vi "Calibration Verfiy new.vi"() -> ()   [LabVIEW 2011]
panel:
  out "error out 2":errorcluster
  out "StatusIsFalse 8":i16
  out "StatusIsFalse 7":i32
  out "StatusIsFalse 3":i16
  out "DONE?":bool
  out "Need More Pwr Reporting":i16
  out "Numeric 2":i32
  out "StatusIsFalse 6":i16
  out "StatusIsFalse 5":i16
  out "StatusIsFalse 4":i16
  out "StatusIsFalse 2":i16
  out "StatusIsFalse":i16
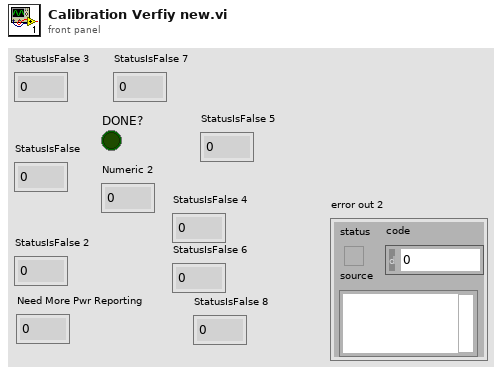
[diagram p1: front panel]
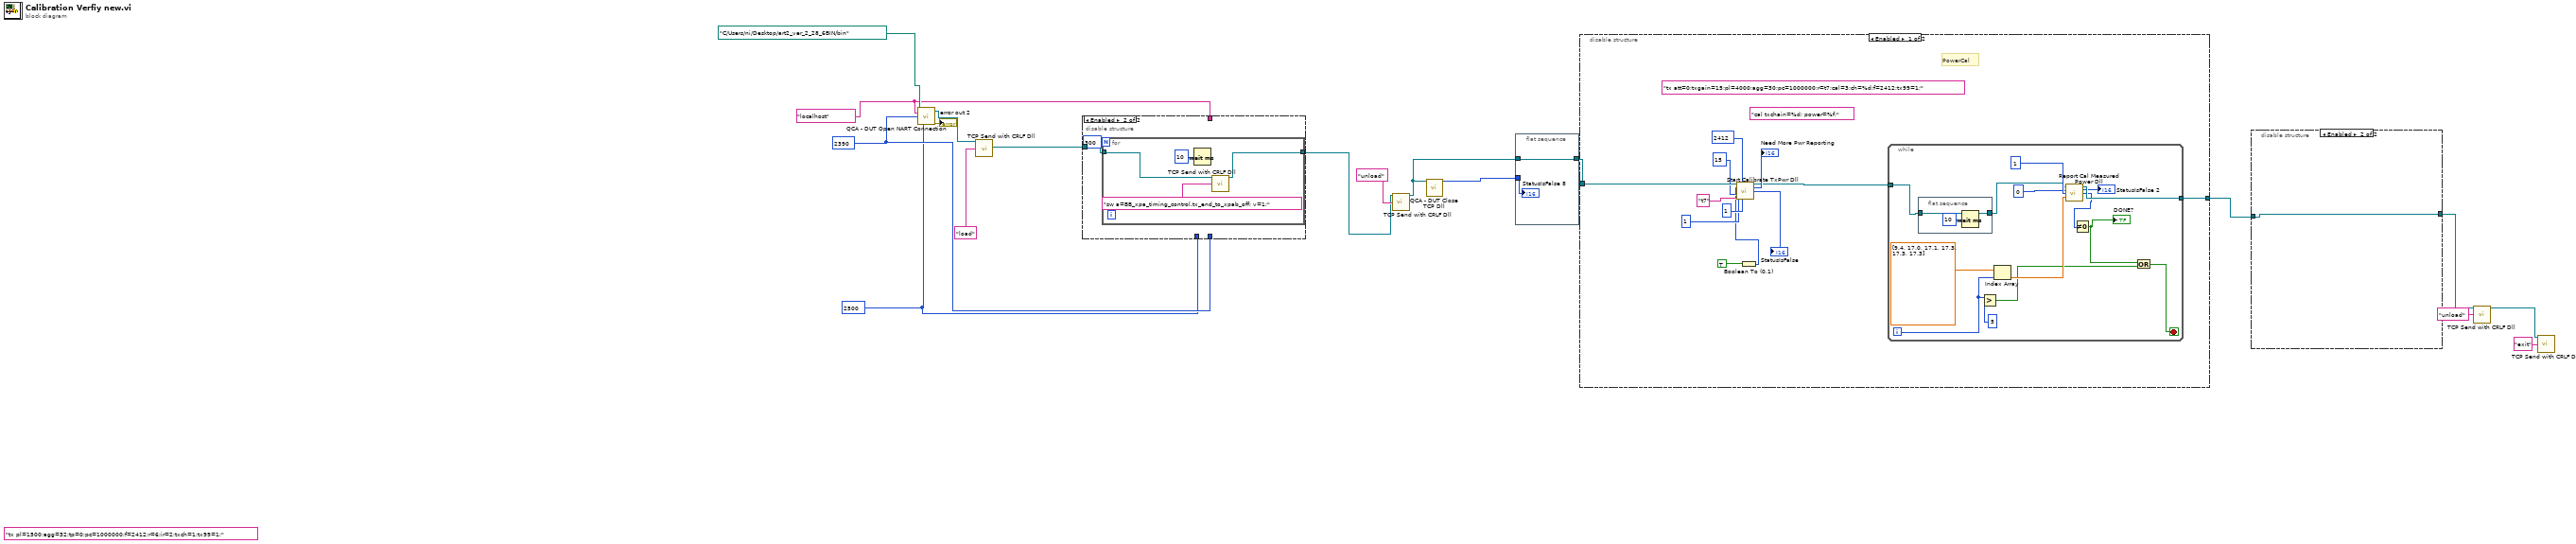
[diagram p0: block diagram]
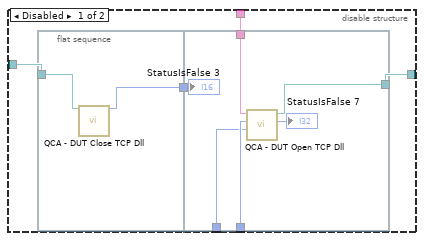
[diagram p2: hidden frame]
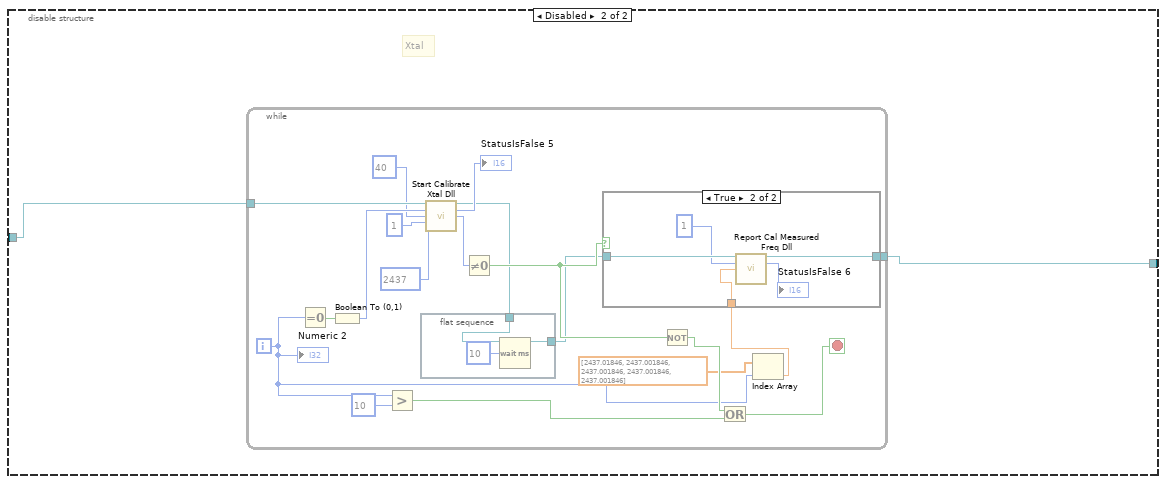
[diagram p3: hidden frame]
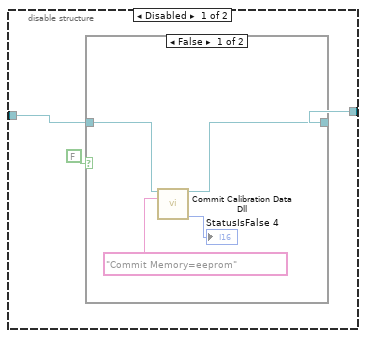
[diagram p5: hidden frame]
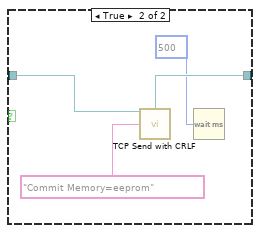
[diagram p6: hidden frame]
diagram:
  (unwired) "tx pl=1500;agg=32;tp=0;pc=1000000;f=2412;r=6;ir=2;txch=1;tx99=1;"
  w9 = 2500 ("Timeout (2500ms)")
  w10 = u32 2390 ("port (2390)")
  w11 = "localhost" ("IP Address (\"\": localhost)")
  n1 = call "QCA - DUT Open NART Connection.vi"("NART Directory"=path "C:/Users/ni/Desktop/art2_ver_2_28_6BIN/bin", "IP Address (\"\": localhost)"=w11, "port (2390)"=w10, "Timeout (2500ms)"=w9) -> ("NART TCP Connection"=w17:refnum<k5>, "error out"=→"error out 2":errorcluster)  [unwired: 10 in]
  n2 = call "TCP Send with CRLF Dll.vi"("CART TCP Connection"=w17, "CommandIn"="load") -> ("CART TCP Connection Out"=w4:refnum<k5>)  [unwired: 13 in]
  n3 = disable-structure shown="Enabled" {
    disable-tunnel: w4 -> [w23 w35]
    disable-tunnel: w11 -> [w22 _]
    disable-tunnel: w10 -> [w21 _]
    disable-tunnel: w9 -> [w20 _]
    disable-tunnel: [w19 w34] -> w1
    frame Disabled {
      n4 = flat-sequence {
        tunnel: w23 -> [w26]
        tunnel: [w25] -> w24
        tunnel: w22 -> [w32]
        tunnel: w21 -> [w31]
        tunnel: w20 -> [w30]
        tunnel: [w29] -> w19
        tunnel: w24 -> [w28]
        frame #0 {
          n5 = call "QCA - DUT Close TCP Dll.vi"("CART TCP Connection"=w26) -> ("StatusIsFalse"=w25:i16)  [unwired: 14 in]
        }
        frame #1 {
          n6 = call "QCA - DUT Open TCP Dll.vi"("Timeout (2500ms)"=w30, "port (2390)"=w31, "IP Address (\"\": localhost)"=w32) -> ("StatusIsFalse"=→"StatusIsFalse 7":i32, "NART TCP Connection"=w29:refnum<k5>)  [unwired: 7 in]
          "StatusIsFalse 3" <- w28
        }
      }
    }
    frame Enabled {
      n7 = for {
        N: 300 -> [_]
        tunnel: w35 -> [w39]
        tunnel: [w38] -> w34
        n8 = Wait (ms)(milliseconds to wait=u32 10) -> ()  [unwired: 1 out]
        n9 = call "TCP Send with CRLF Dll.vi"("CART TCP Connection"=w39, "CommandIn"="sw a=BB_xpa_timing_control.tx_end_to_xpab_off; v=1;") -> ("CART TCP Connection Out"=w38:refnum<k5>)  [unwired: 13 in]
      }
    }
  }
  n10 = call "TCP Send with CRLF Dll.vi"("CART TCP Connection"=w1, "CommandIn"="unload") -> ("CART TCP Connection Out"=w3:refnum<k5>)  [unwired: 13 in]
  n11 = call "QCA - DUT Close TCP Dll.vi"("CART TCP Connection"=w3) -> ("StatusIsFalse"=w7:i16)  [unwired: 14 in]
  n12 = flat-sequence {
    tunnel: w3 -> [w41]
    tunnel: [w41] -> w8
    tunnel: w7 -> [w40]
    frame #0 {
      "StatusIsFalse 8" <- w40
    }
  }
  n13 = disable-structure shown="Enabled" {
    disable-tunnel: w8 -> [w53 w71]
    disable-tunnel: [w52 w70] -> w16
    frame Enabled {
      (unwired) "cal txchain=%d; power=%f;" ("Name")
      (unwired) "tx att=0;txgain=15;pl=4000;agg=30;pc=1000000;r=t7;cal=3;ch=%d;f=2412;tx99=1;" ("Name")
      # "PowerCal"
      n14 = Boolean To (0,1)(Boolean=TRUE) -> (0, 1=w45:i16)
      n15 = call "Start Calibrate TxPwr Dll.vi"("CART TCP Connection In"=w53, "TxPwrCalFreq"=2412, "Need Send Cal Command"=w45, "isFirstFreq"=u8 1, "TxPwrCalGain"=u32 15, "TxPwrCalRate"="t7", "TxPwrCalCh"=u32 1) -> ("CART TCP Connection Out"=w42:refnum<k5>, "Need More Pwr Reporting"=→"Need More Pwr Reporting":i16, "StatusIsFalse"=→"StatusIsFalse":i16)  [unwired: 6 in]
      n16 = while {
        tunnel: [w67] -> w52
        tunnel: w42 -> [w58]
        i -> [w56]
        stop <- w59 stop-if-true
        n17 = flat-sequence {
          tunnel: w58 -> [w69]
          tunnel: [w69] -> w57
          frame #0 {
            n18 = Wait (ms)(milliseconds to wait=u32 10) -> ()  [unwired: 1 out]
          }
        }
        n19 = Greater?(x=w56, y=5) -> (0:w62:bool)
        n20 = Index Array(array=dbl[] [9.4, 17.0, 17.1, 17.3, 17.3, 17.3], index=w56) -> (element=w63:dbl)
        n21 = call "Report Cal Measured Power Dll.vi"("CART TCP Connection In"=w57, "LastFreqCommit"=u8 0, "TxPwrCalChain"=u32 1, "TxPwrCalVal"=w63) -> ("CART TCP Connection Out"=w67:refnum<k5>, "StatusIsFalse"=→"StatusIsFalse 2":i16, "DONE?"=w55:i16)  [unwired: 9 in]
        n22 = Not Equal To 0?(x=w55) -> (x != 0?=w54:bool)
        "DONE?" <- w54
        n23 = Or(x=w54, y=w62) -> (x .or. y?=w59:bool)
      }
    }
    frame Disabled {
      # "Xtal"
      n24 = while {
        tunnel: w71 -> [w90]
        tunnel: [w82] -> w70
        i -> [w73]
        stop <- w77 stop-if-true
        n25 = Equal To 0?(x=w73) -> (x = 0?=w89:bool)
        n26 = Boolean To (0,1)(Boolean=w89) -> (0, 1=w88:i16)
        n27 = Greater?(x=w73, y=10) -> (0:w78:bool)
        n28 = flat-sequence {
          tunnel: [w91] -> w75
          tunnel: w76 -> [w91]
          frame #0 {
            n29 = Wait (ms)(milliseconds to wait=u32 10) -> ()  [unwired: 1 out]
          }
        }
        n30 = call "Start Calibrate Xtal Dll.vi"("CART TCP Connection In"=w90, "Need Send Cal Command"=w88, "XtalCalGain"=u32 40, "XtalCalCh"=u32 1, "XtalCalFreq"=2437) -> ("CART TCP Connection Out"=w76:refnum<k5>, "StatusIsFalse"=→"StatusIsFalse 5":i16, "Need More Freq Reporting"=w83:i16)  [unwired: 8 in]
        n31 = Not Equal To 0?(x=w83) -> (x != 0?=w81:bool)
        n32 = Not(x=w81) -> (.not. x?=w79:bool)
        n33 = Or(x=w79, y=w78) -> (x .or. y?=w77:bool)
        n34 = Index Array(array=dbl[] [2437.01846, 2437.001846, 2437.001846, 2437.001846, 2437.001846], index=w73) -> (element=w72:dbl)
        n35 = case shown="True" w81 {
          tunnel: w75 -> [w93 w98]
          tunnel: [w93 w95] -> w82
          tunnel: w72 -> [_ w94]
          frame False {
          }
          frame True {
            n36 = call "Report Cal Measured Freq Dll.vi"("CART TCP Connection In"=w98, "XtalCalChain"=u32 1, "XtalCalVal"=w94) -> ("CART TCP Connection Out"=w95:refnum<k5>, "StatusIsFalse"=→"StatusIsFalse 6":i16)  [unwired: 11 in]
          }
        }
        "Numeric 2" <- w73
      }
    }
  }
  n37 = disable-structure shown="Enabled" {
    disable-tunnel: w16 -> [w101 w110]
    disable-tunnel: [w100 w110] -> w15
    frame Disabled {
      n38 = case shown="False" FALSE {
        tunnel: w101 -> [w105 w109]
        tunnel: [w104 w108] -> w100
        frame False {
          n39 = call "Commit Calibration Data Dll.vi"("CART TCP Connection In"=w105, "CommitMemory"="Commit Memory=eeprom") -> ("CART TCP Connection Out"=w104:refnum<k5>, "StatusIsFalse"=→"StatusIsFalse 4":i16)  [unwired: 12 in]
        }
        frame True {
          n40 = call "TCP Send with CRLF.vi"("CART TCP Connection"=w109, "data in"="Commit Memory=eeprom") -> ("CART TCP Connection Out"=w108:refnum<k5>)  [unwired: 12 in, 1 out]
          n41 = Wait (ms)(milliseconds to wait=u32 500) -> ()  [unwired: 1 out]
        }
      }
    }
    frame Enabled {
    }
  }
  n42 = call "TCP Send with CRLF Dll.vi"("CART TCP Connection"=w15, "CommandIn"="unload") -> ("CART TCP Connection Out"=w13:refnum<k5>)  [unwired: 13 in]
  n43 = call "TCP Send with CRLF Dll.vi"("CART TCP Connection"=w13, "CommandIn"="exit") -> ()  [unwired: 13 in, 1 out]
